vi "Wrap index.vi"(10 "Index":i32, 11 "Size":i32) -> ()   [LabVIEW 2020]
panel:
  in  "Jumps":i32
  out "Index Out":i32
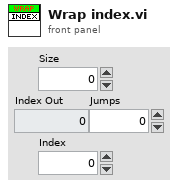
[diagram p1: front panel]
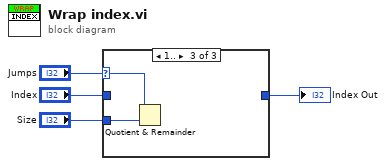
[diagram p0: block diagram]
diagram:
  n1 = case shown="1.." "Jumps" {
    selector: "Jumps" -> [_ _ w6]
    tunnel: "Index" -> [w5 _ _]
    tunnel: "Size" -> [_ _ w7]
    tunnel: [w5 _ _] -> w2
    frame 0 {
    }
    frame ..-1 {
    }
    frame 1.. {
      n2 = Quotient & Remainder(x=w6, y=w7) -> ()  [unwired: 2 out]
    }
  }
  "Index Out" <- w2
